vi "Calibragem.vi"() -> ()   [LabVIEW 2013]
panel:
  in  "Iniciar":bool
  in  "Calibragem":string[][](table)=[["", "1", "2", "3", "4"], ["Base", "BC", "BC", "BR", "BR"], ["Estado", "1", "0", "1", "0"], ["Amostra", "5", "5", "5", "5"]]
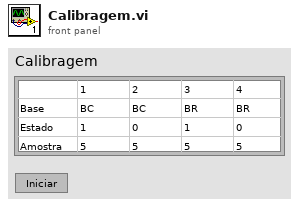
[diagram p1: front panel]
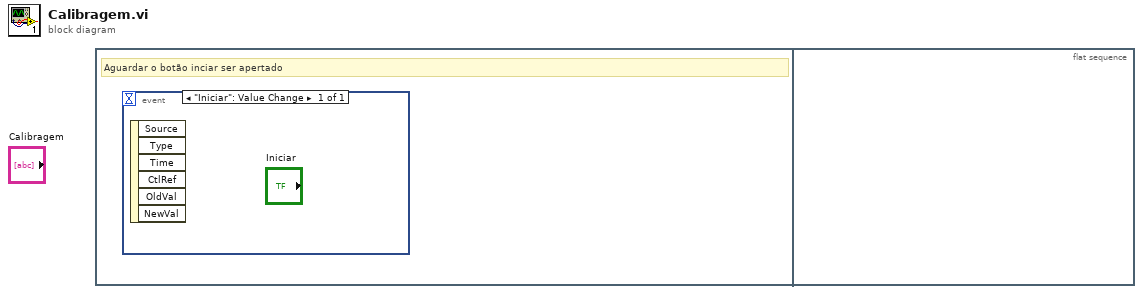
[diagram p0: block diagram]
diagram:
  n1 = flat-sequence {
    frame #0 {
      # "Aguardar o botão inciar ser apertado"
      n2 = event shown="[0] \"Iniciar\": Value Change" {
        selector: _ -> [_]
        dyn-events: _ -> [_]
        timeout: _ -> [_]
        event "Iniciar": Value Change {
          n3 = event-data() -> ()  [unwired: 1 in, 6 out]
        }
      }
    }
    frame #1 {
    }
  }
